vi "FlushExitTest.vi"(8 "error in (no error)":errorcluster, 9 "SeqExeQuueIn":refnum<queue>, 11 "TestSeqClass in":refnum<class "TestSeqClass.lvclass">) -> (0 "error out":errorcluster, 3 "TestSeqClass out":refnum<class "TestSeqClass.lvclass">)   [LabVIEW 2019, in "TestSeqClass.lvclass"]
uses:
  TestSeqClass.lvclass
  GUIHandler_Main/GUI_Handler_Main.lvclass
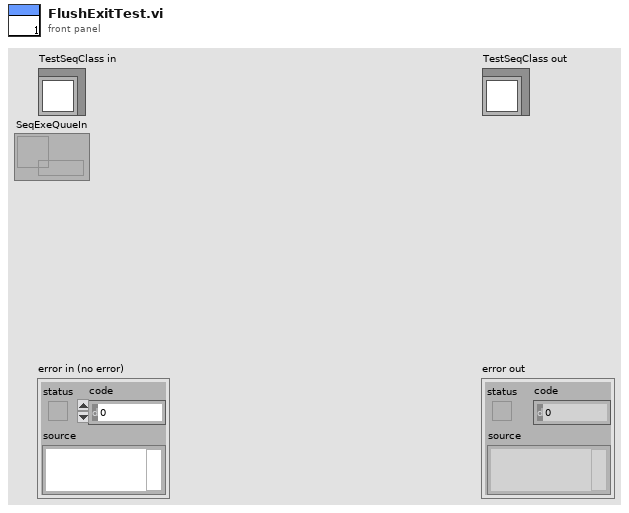
[diagram p1: front panel]
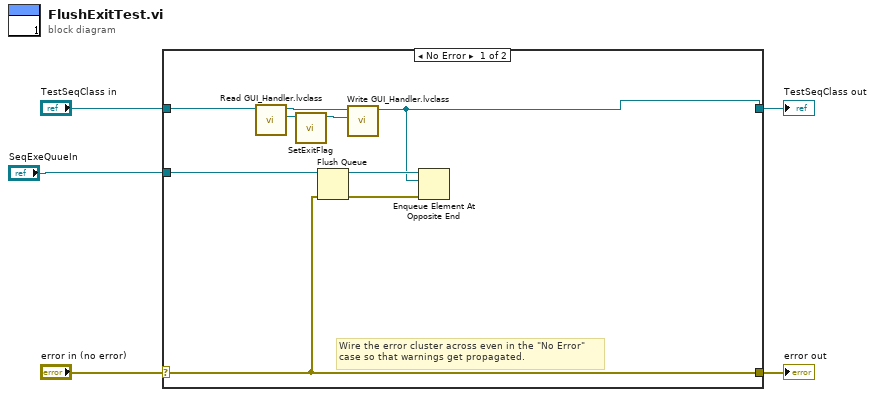
[diagram p0: block diagram]
diagram:
  n1 = case shown="No Error" "error in (no error)" {
    selector: "error in (no error)" -> [w13 w16]
    tunnel: [w13 w16] -> w4
    tunnel: [w6 w15] -> w2
    tunnel: "TestSeqClass in" -> [w10 w15]
    tunnel: "SeqExeQuueIn" -> [w14 _]
    frame No Error {
      # "Wire the error cluster across even in the \"No Error\"\ncase so that warnings get propagated."
      n2 = call-dynamic "Read GUI_Handler.lvclass.vi"("TestSeqClass in"=w10) -> ("GUI_Handler.lvclass"=w9:refnum<class "GUI_Handler_Main.lvclass">, "TestSeqClass out"=w7:refnum<class "TestSeqClass.lvclass">)  [unwired: 8 in, 1 out]
      n3 = call "SetExitFlag.vi"("GUI_Handler_Main in"=w9) -> ("GUI_Handler_Main out"=w8:refnum<class "GUI_Handler_Main.lvclass">)  [unwired: 9 in, 1 out]
      n4 = Flush Queue(queue=w14, error in (no error)=w13) -> (queue out=w12:refnum<queue>, error out=w11:errorcluster)  [unwired: 1 out]
      n5 = call-dynamic "Write GUI_Handler.lvclass.vi"("GUI_Handler.lvclass"=w8, "TestSeqClass in"=w7) -> ("TestSeqClass out"=w6:refnum<class "TestSeqClass.lvclass">)  [unwired: 8 in, 1 out]
      n6 = Enqueue Element At Opposite End(queue=w12, element=w6, error in (no error)=w11) -> ()  [unwired: 1 in, 3 out]
    }
    frame Error {
    }
  }
  "error out" <- w4
  "TestSeqClass out" <- w2
